vi "Destroy.vi"(8 "error in (no error)":errorcluster) -> (0 "error out":errorcluster)   [LabVIEW 2026, in "TALOS.lvlib" / "Classes.lvlib" / "Error Filter.lvclass"]
doc: "Use this VI to add an error to be skipped in the future. If repetitions and time are both left to zero, the error will be permanently skipped: otherwise the error will be skipped until at least one of the two conditions will be met."
uses:
  Error Filter.lvclass
  Ancestor/Ancestor/Ancestor.lvclass/Ancestor.ctl
  Support VIs/Generate Error.vi
  FGV/Error Memory/Get Error Description.vi
  Support VIs/Get PC name.vi
  Ancestor/Ancestor/Read ID.vi
  Support VIs/Get Class Name.vi
  <vilib>/Utility/error.llb/Clear Errors.vi
  FGV/Error Memory/Error Memory Core.vi
  <vilib>/AdvancedString/Delimited String to 1D String Array.vi
  <vilib>/AdvancedString/Delimited String to 1D String Array (string).vi
  Support VIs/Circus Root Path.vi
  FGV/Error Memory/Error Crt Lvl checker.vi
  FGV/Error Memory/Error Memory Core.vi/40c8088d-b597-4017-91af-faa98e00292e.vi
  FGV/Error Memory/Error Memory Core.vi/d4a3ab98-063c-4e44-b43d-fbdcfe6c2be2.vi
  Support VIs/Global Memory.vi
  <vilib>/Utility/LVClass/Get LV Class Name.vi
  Support VIs/Is in Packed Library.vi
  Support VIs/TALOS Root path.vi
  Support VIs/Read CSV worksheet.vi
  Support VIs/Global Constants.vi
  <vilib>/Utility/error.llb/General Error Handler.vi
  Support VIs/Error Log.vi
  Ancestor/Ancestor/Ancestor.lvclass
  <vilib>/Comparison/Equal/Equal Functor/Equal Functor.lvclass
  TALOS.lvlib
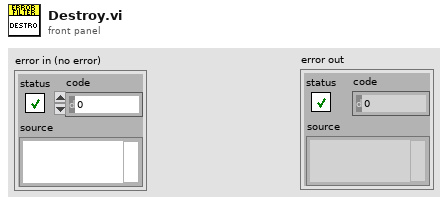
[diagram p1: front panel]
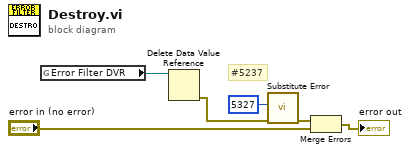
[diagram p0: block diagram]
diagram:
  # "#5237"
  n1 = global read "Global Memory.vi" "Error Filter DVR"() -> (w6:refnum<data-value>)
  n2 = Delete Data Value Reference(data value reference=w6) -> (error out=w3:errorcluster)  [unwired: 1 in, 1 out]
  n3 = call "Substitute Error.vi"("error in (no error)"=w3, "Error Code"=5327) -> ("error out"=w2:errorcluster)  [unwired: 9 in]
  n4 = Merge Errors(w2, "error in (no error)") -> (→"error out":errorcluster)
